vi "ProbingTestAuto.vi"() -> ()   [LabVIEW 2018]
uses:
  <vilib>/Utility/file.llb/Read Delimited Spreadsheet (DBL).vi
  <vilib>/Utility/file.llb/Read Delimited Spreadsheet (I64).vi
panel:
  in  "Sensor":string(combo)="R0Hamamatsu"
  in  "Camera Offset Y":dbl=1.7
  in  "Camera Offset X":dbl=-98.89
  in  "Begin":bool
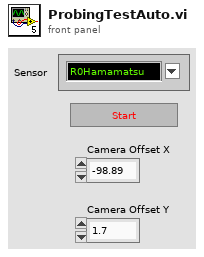
[diagram p1: front panel]
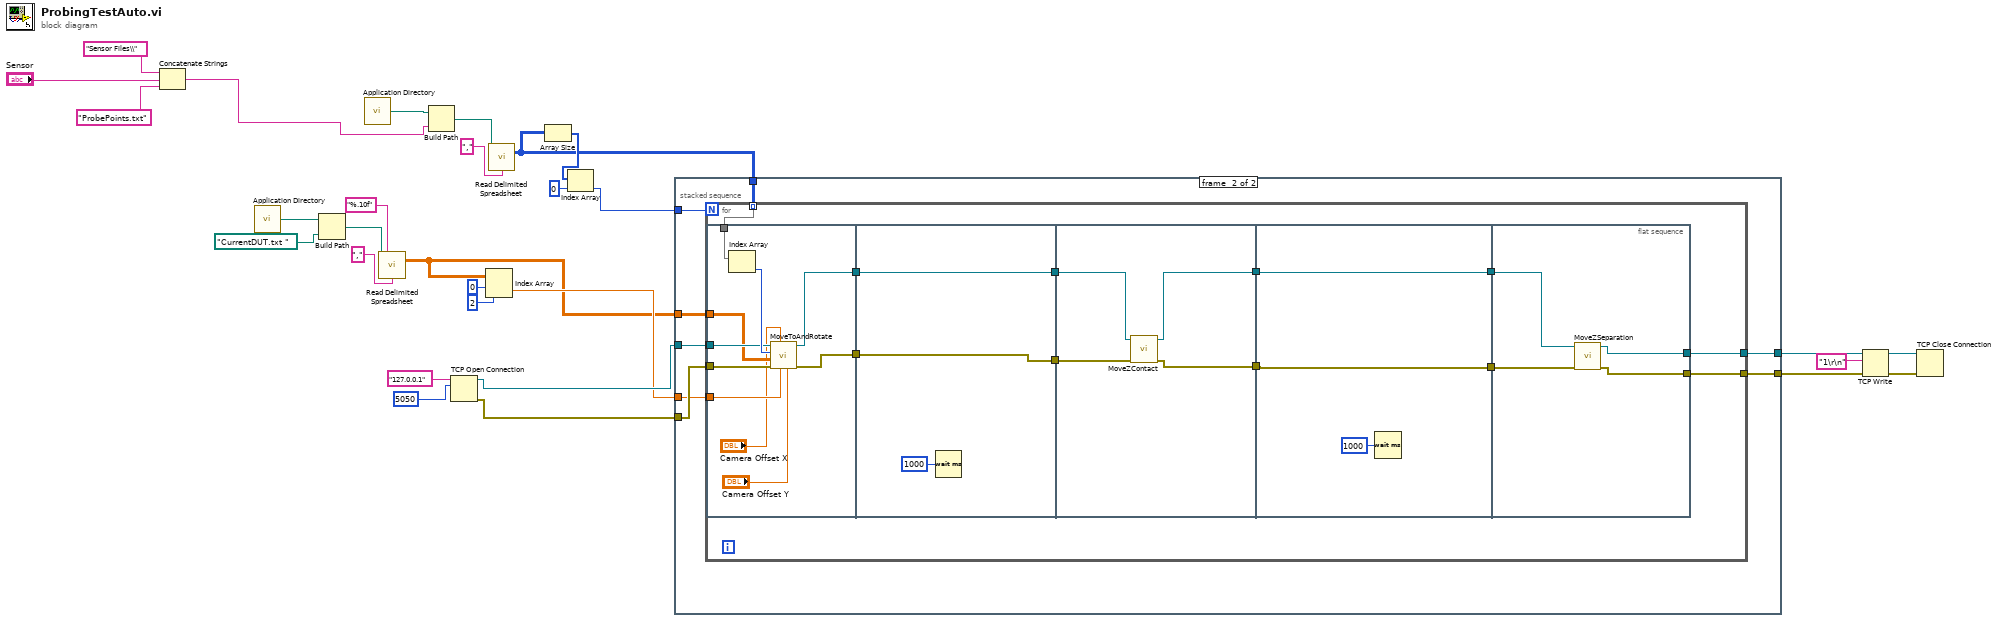
[diagram p0: block diagram]
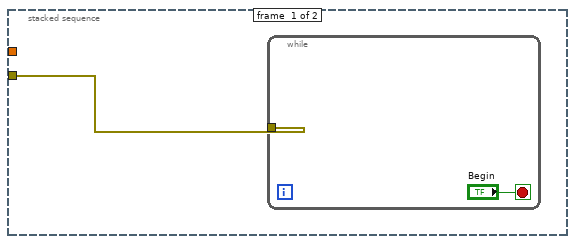
[diagram p2: hidden frame]
diagram:
  n1 = Concatenate Strings("Sensor Files\\" ("string"), "Sensor", "ProbePoints.txt" ("string")) -> (w1:string)
  n2 = call <vilib>:"Application Directory.vi"() -> ("Application Directory"=w26:path)
  n3 = Build Path(base path=w26, name or relative path=path "CurrentDUT.txt " ("file path (dialog if empty)")) -> (appended path=w27:path)
  n4 = call <vilib>:"Application Directory.vi"() -> ("Application Directory"=w6:path)
  n5 = call-poly <vilib>:"Read Delimited Spreadsheet.vi"("file path (dialog if empty)"=w27, "format (%.3f)"="%.10f", "delimiter (\\t)"="," ("delimiter (\\t)")) -> ("all rows"=w12:dbl[][])  [unwired: 7 in, 5 out]
  n6 = Build Path(base path=w6, name or relative path=w1) -> (appended path=w21:path)
  n7 = TCP Open Connection(address="127.0.0.1", remote port or service name=u16 5050) -> (connection ID=w14:refnum<k5>, error out=w5:errorcluster)  [unwired: 3 in]
  n8 = Index Array(array=w12, index (row)=0, index (col)=2 ("disabled index (col)")) -> (element=w13:dbl)
  n9 = call-poly <vilib>:"Read Delimited Spreadsheet.vi"("file path (dialog if empty)"=w21, "delimiter (\\t)"="," ("delimiter (\\t)")) -> ("all rows"=w15:i64[][])  [unwired: 8 in, 5 out]
  n10 = Array Size(array=w15) -> (size(s)=w20:i32[])
  n11 = Index Array(array=w20, index=0) -> (element=w16:i32)
  n12 = stacked-sequence {
    tunnel: w5 -> [w30 w36]
    tunnel: w16 -> [_ w39]
    tunnel: w15 -> [_ w38]
    tunnel: w14 -> [_ w37]
    tunnel: w13 -> [_ w35]
    tunnel: w12 -> [_ w34]
    tunnel: [_ w33] -> w8
    tunnel: [_ w32] -> w7
    frame #0 {
      n13 = while {
        tunnel: w30 -> [_]
        stop <- "Begin" stop-if-true
      }
    }
    frame #1 {
      n14 = for {
        N: w39 -> [_]
        tunnel: w38 -> [w54] mode=indexing
        tunnel: w37 -> [w53]
        tunnel: w36 -> [w52]
        tunnel: w35 -> [w51]
        tunnel: w34 -> [w50]
        tunnel: [w41] -> w33
        tunnel: [w40] -> w32
        n15 = flat-sequence {
          tunnel: w54 -> [w64]
          tunnel: w53 -> [w62]
          tunnel: w52 -> [w61]
          tunnel: w51 -> [w60]
          tunnel: w50 -> [w59]
          tunnel: [w58] -> w49
          tunnel: [w57] -> w48
          tunnel: w49 -> [w65]
          tunnel: w48 -> [w66]
          tunnel: [w66] -> w47
          tunnel: [w65] -> w46
          tunnel: w47 -> [w71]
          tunnel: w46 -> [w70]
          tunnel: [w69] -> w45
          tunnel: [w68] -> w43
          tunnel: w45 -> [w74]
          tunnel: [w73] -> w44
          tunnel: w43 -> [w73]
          tunnel: [w74] -> w42
          tunnel: w44 -> [w78]
          tunnel: w42 -> [w77]
          tunnel: [w76] -> w41
          tunnel: [w75] -> w40
          frame #0 {
            n16 = Index Array(array=w64) -> (element=w63:i64)  [unwired: 1 in]
            n17 = call "MoveToAndRotate.vi"("Camera Offset Y"="Camera Offset Y", "Initial Angle"=w60, "Camera Offset X"="Camera Offset X", "Error In"=w61, "Probing Array"=w59, "Probe Index"=w63, "connection ID"=w62) -> ("error out"=w58:errorcluster, "connection ID 2"=w57:refnum<k5>)  [unwired: 3 in]
          }
          frame #1 {
            n18 = Wait (ms)(milliseconds to wait=u32 1000) -> ()  [unwired: 1 out]
          }
          frame #2 {
            n19 = call "MoveZContact.vi"("error in (no error) 2"=w70, "connection ID 2"=w71) -> ("error out"=w69:errorcluster, "connection ID"=w68:refnum<k5>)  [unwired: 8 in]
          }
          frame #3 {
            n20 = Wait (ms)(milliseconds to wait=u32 1000) -> ()  [unwired: 1 out]
          }
          frame #4 {
            n21 = call "MoveZSeparation.vi"("error in (no error) 2"=w77, "connection ID 2"=w78) -> ("error out"=w75:errorcluster, "connection ID"=w76:refnum<k5>)  [unwired: 8 in]
          }
        }
      }
    }
  }
  n22 = TCP Write(connection ID=w8, data in="1\r\n", error in (no error)=w7) -> (connection ID out=w10:refnum<k5>, error out=w11:errorcluster)  [unwired: 1 in, 1 out]
  n23 = TCP Close Connection(connection ID=w10, error in (no error)=w11) -> ()  [unwired: 1 in, 2 out]
